vi "Taskkill.vi"(8 "error in (no error)":errorcluster) -> (0 "error out":errorcluster, 2 "python was stopped?":bool)   [LabVIEW 2024]
doc: "Stop analysis immediately by stopping python script running. Delete all features found for current image to avoid duplicates in future."
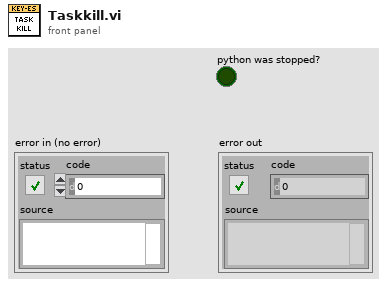
[diagram p1: front panel]
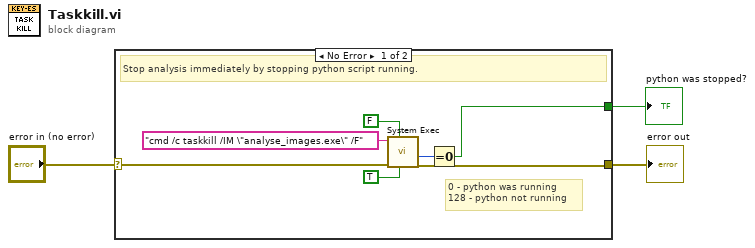
[diagram p0: block diagram]
diagram:
  n1 = case shown="No Error" "error in (no error)" {
    selector: "error in (no error)" -> [w7 w11]
    tunnel: [w6 w11] -> w3
    tunnel: [w4 _] -> w1
    frame No Error {
      # "0 - python was running\n128 - python not running"
      # "Stop analysis immediately by stopping python script running."
      n2 = call <vilib>:"System Exec.vi"("run minimized? (F)"=TRUE, "wait until completion? (T)"=FALSE, "error in (no error)"=w7, "command line"="cmd /c taskkill /IM \"analyse_images.exe\" /F") -> ("error out"=w6:errorcluster, "return code"=w5:i32)  [unwired: 4 in, 2 out]
      n3 = Equal To 0?(x=w5) -> (x = 0?=w4:bool)
    }
    frame Error {
    }
  }
  "error out" <- w3
  "python was stopped?" <- w1
